vi "Read (Waveform).vi"(8 "error in (no error)":errorcluster, 9 "Timeout (10000 ms)":u32=10000, 10 "Source (0: Channel 1)":u16(ring) items=["Channel 1", "Channel 2", "Channel 3", "Channel 4", "Math", "Reference A", "Reference B", "Reference C", "Reference D", "FFT"], 11 "TDS 2000 in":refnum<class "TDS 2000.lvclass">) -> (0 "error out":errorcluster, 2 "Waveform Data":waveform(dbl)(graph), 3 "TDS 2000 out":refnum<class "TDS 2000.lvclass">)   [LabVIEW 2020, in "Oscilloscope.lvlib" / "TDS 2000.lvclass"]
uses:
  TDS 2000.lvclass
  C:/Users/ronad/Osciloscopio/Osciloscopio DQMH/Libraries/Oscilloscope/Clases/Osciloscopio/Osciloscopio.lvclass
  Osciloscopio/Osciloscopio.lvclass/Osciloscopio.ctl
  Osciloscopio/Read COM.vi
  Osciloscopio/Write COM.vi
  <instrlib>/Tektronix TDS 200 1000 2000 Series/Public/Data/Read (Single Waveform).vi
  <instrlib>/Tektronix TDS 200 1000 2000 Series/Tektronix TDS 200 1000 2000 Series.lvlib
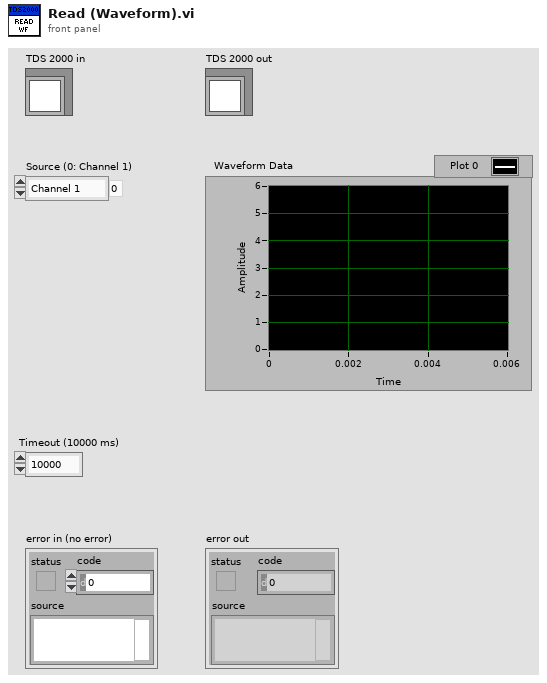
[diagram p1: front panel]
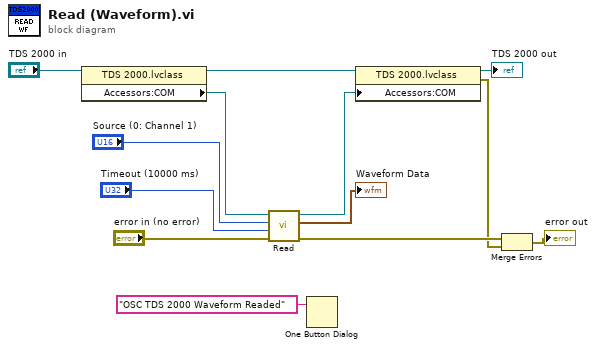
[diagram p0: block diagram]
diagram:
  n1 = property class="TDS 2000.lvclass"(reference="TDS 2000 in") -> (reference out=w11:refnum<class "TDS 2000.lvclass">, "Accessors:COM"=w12:refnum<visa-resource-name>)  [unwired: 1 in, 1 out]
  n2 = call-poly <instrlib>:"Read.vi"("error in (no error)"="error in (no error)", "Timeout (10000 ms)"="Timeout (10000 ms)", "Source (0: Channel 1)"="Source (0: Channel 1)", "VISA resource name"=w12) -> ("error out"=w5:errorcluster, "Waveform Data"=→"Waveform Data":waveform(dbl), "VISA resource name out"=w10:refnum<visa-resource-name>)  [unwired: 5 in]
  n3 = One Button Dialog(message="OSC TDS 2000 Waveform Readed") -> ()  [unwired: 1 in, 1 out]
  n4 = property class="TDS 2000.lvclass"(reference=w11, "Accessors:COM"=w10) -> (reference out=→"TDS 2000 out":refnum<class "TDS 2000.lvclass">, error out=w2:errorcluster)  [unwired: 1 in]
  n5 = Merge Errors(w5, w2) -> (→"error out":errorcluster)
